vi "Union Unified Msg Set.vi"(7 "Actor":refnum<class "Actor.lvclass">, 10 "Unified Msg Set in":T1) -> (2 "Unified Msg Set out":T1)   [LabVIEW 2025, in "jettl.lvlib"]
uses:
  jettl.lvlib
  Actor/Msg Set.ctl
  Msg/Msg.lvclass
  Actor/Actor/Actor.lvclass
  Actor/Actor.lvlib
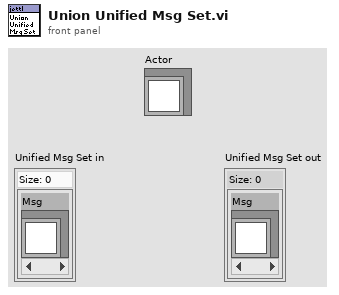
[diagram p1: front panel]
types:
  T1 = typedef "jettl.lvlib/Actor.lvlib/Msg Set.ctl" = set{refnum<class "Msg.lvclass">}
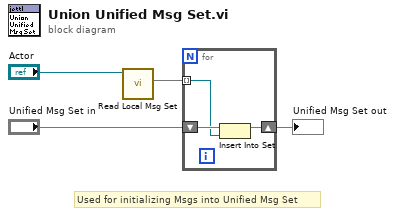
[diagram p0: block diagram]
diagram:
  # "Used for initializing Msgs into Unified Msg Set"
  n1 = call-dynamic "Read Local Msg Set.vi"("Actor in"="Actor") -> ("Local Msg Set"=w3:T1)  [unwired: 10 in]
  n2 = for {
    shift-right: [w6] -> w4
    shift-left: "Unified Msg Set in" -> [w7]
    tunnel: w3 -> [w5] mode=indexing
    n3 = Insert Into Set(10:w5, 11:w7) -> (3:w6:T1)  [unwired: 1 out]
  }
  "Unified Msg Set out" <- w4
